vi "Get Menu Launch Info__jki_lib_application_control -- VI Tester.vi"(8 "error in (no error)":errorcluster) -> (0 "error out":errorcluster, 2 "Menu Launch info":T1)   [LabVIEW 2011]
doc: "Returns menu-launch info, including selected project items."
uses:
  Menu Launch Info - Cluster__jki_lib_application_control -- VI Tester.ctl
  Project Item Info - Cluster__jki_lib_application_control -- VI Tester.ctl
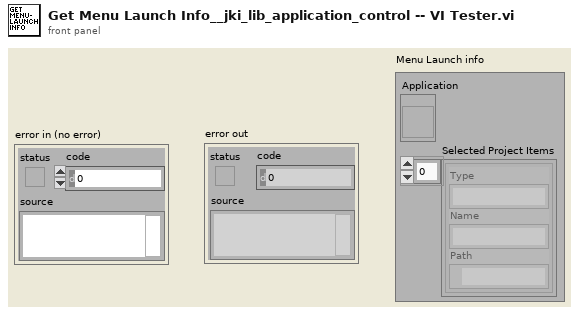
[diagram p1: front panel]
types:
  T1 = typedef "Menu Launch Info - Cluster__jki_lib_application_control -- VI Tester.ctl" = cluster{"Application":refnum<vi>, "Selected Project Items":T2[]}
  T2 = typedef "Project Item Info - Cluster__jki_lib_application_control -- VI Tester.ctl" = cluster{"Type":string, "Name":string, "Path":path}
  T3 = cluster{"App.DefaultApplication":refnum<vi>, "Selected Project Items":T2[]}
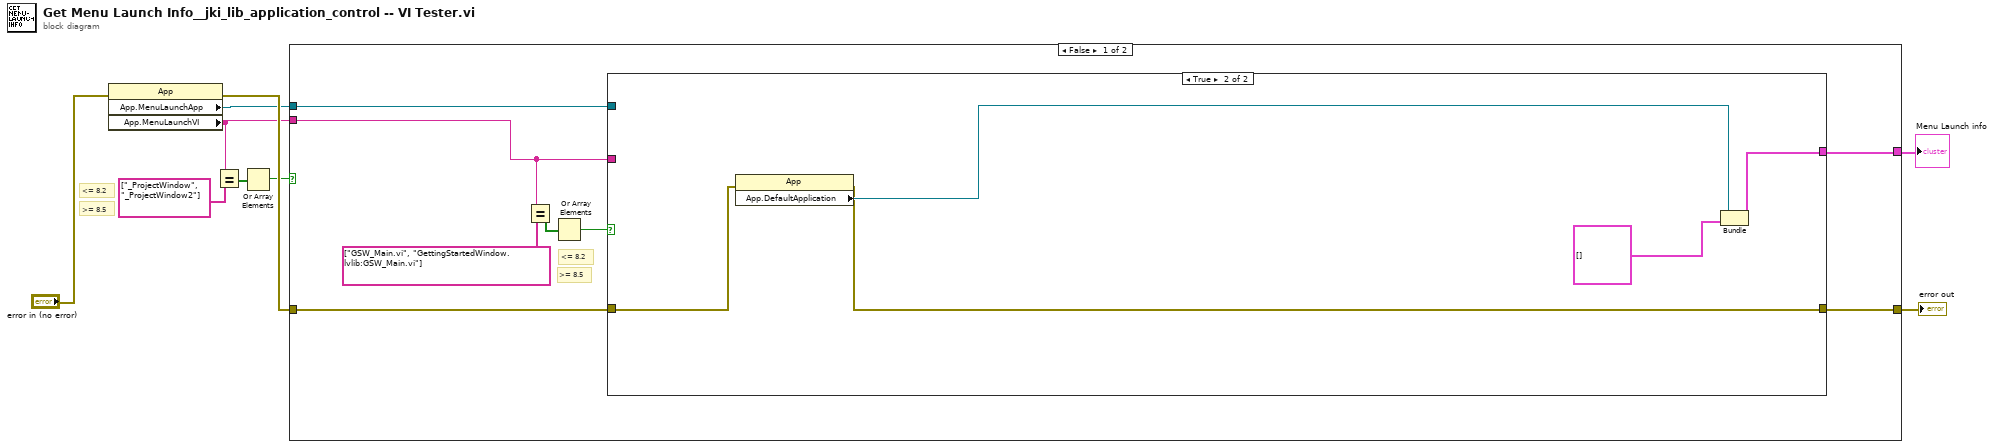
[diagram p0: block diagram]
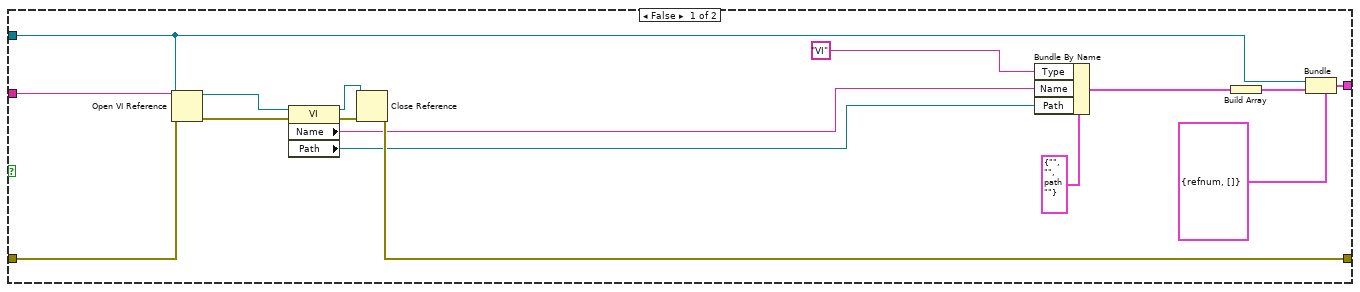
[diagram p2: hidden frame]
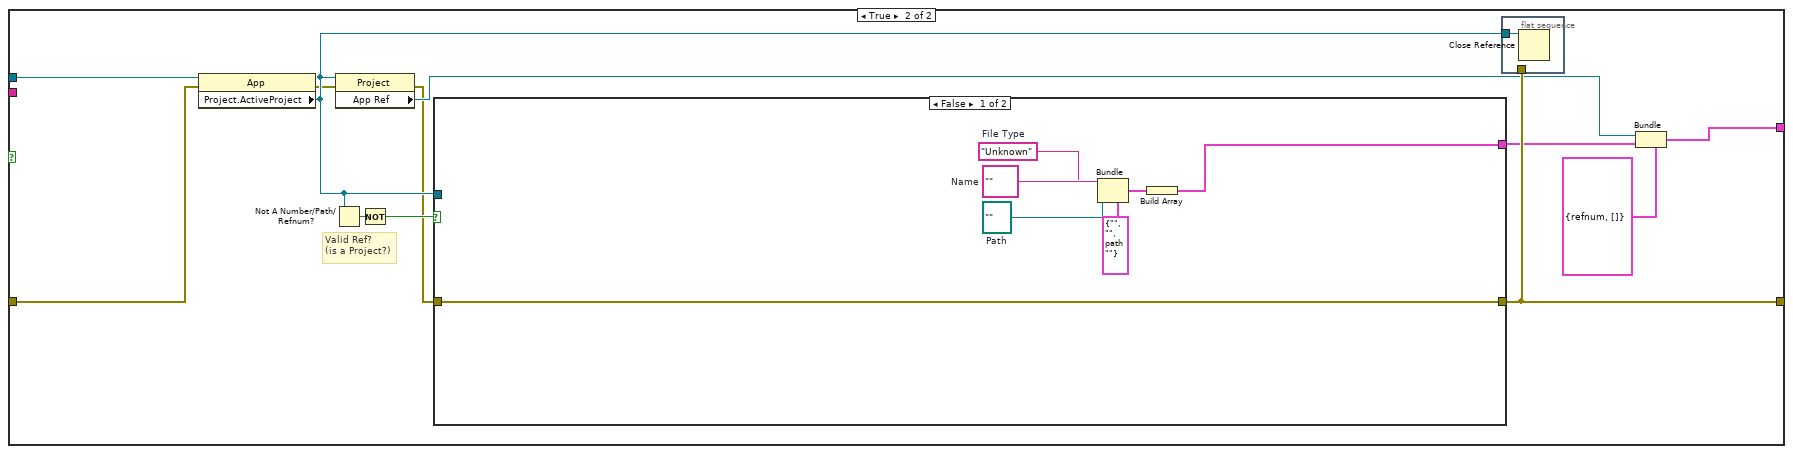
[diagram p3: hidden frame]
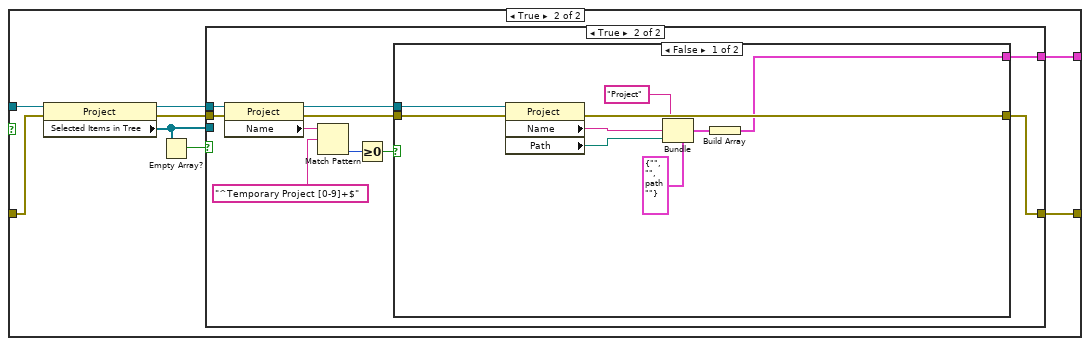
[diagram p4: hidden frame]
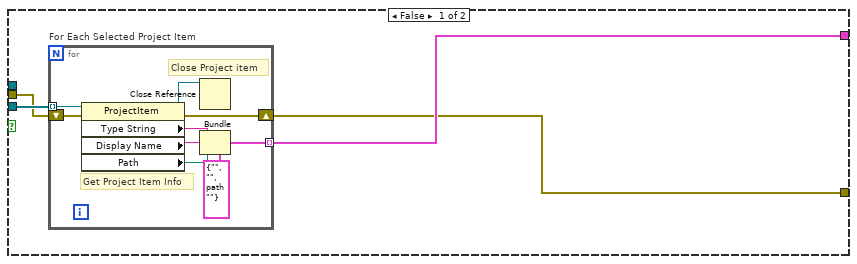
[diagram p5: hidden frame]
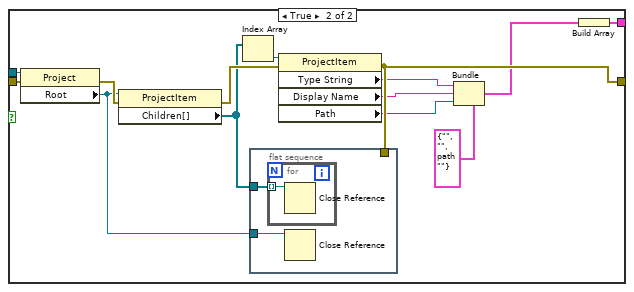
[diagram p6: hidden frame]
diagram:
  # "<= 8.2"
  # ">= 8.5"
  n1 = property class="App"(error in="error in (no error)") -> (error out=w9:errorcluster, "App.MenuLaunchApp"=w8:refnum<vi>, "App.MenuLaunchVI"=w4:string)  [unwired: 1 in, 1 out]
  n2 = Equal?(x=w4, y=string[] ["_ProjectWindow", "_ProjectWindow2"]) -> (x = y?=w2:bool[])
  n3 = Or Array Elements(Boolean array=w2) -> (logical OR=w1:bool)
  n4 = case shown="False" w1 {
    tunnel: w9 -> [w17 w50]
    tunnel: w8 -> [w15 w49]
    tunnel: [w14 w44] -> w7
    tunnel: [w16 w46] -> w6
    tunnel: w4 -> [w13 _]
    frame False {
      # "<= 8.2"
      # ">= 8.5"
      n5 = Equal?(x=w13, y=string[] ["GSW_Main.vi", "GettingStartedWindow.lvlib:GSW_Main.vi"]) -> (x = y?=w12:bool[])
      n6 = Or Array Elements(Boolean array=w12) -> (logical OR=w10:bool)
      n7 = case shown="True" w10 {
        tunnel: w17 -> [w29 w36]
        tunnel: [w28 w35] -> w16
        tunnel: w15 -> [w26 _]
        tunnel: [w25 w38] -> w14
        tunnel: w13 -> [w22 _]
        frame False {
          n8 = Open VI Reference(application reference (local)=w26, vi path=w22, error in (no error)=w29) -> (vi reference=w32:refnum<vi>, error out=w33:errorcluster)  [unwired: 3 in]
          n9 = property class="VI"(reference=w32, error in=w33) -> (reference out=w31:refnum<vi>, error out=w30:errorcluster, "Name"=w21:string, "Path"=w24:path)
          n10 = Close Reference(reference=w31, error in (no error)=w30) -> (error out=w28:errorcluster)
          n11 = Bundle By Name(cluster=T2 {"Type"="", "Name"="", "Path"=path ""} ("Project Item"), "Type"="VI" ("File Type"), "Name"=w21, "Path"=w24) -> (w23:T2)
          n12 = Build Array(w23) -> (w27:T2[])
          n13 = Bundle(cluster=T1 {"Application"=refnum, "Selected Project Items"=[]} ("Menu Launch info"), "Application"=w26, "Selected Project Items"=w27) -> (w25:T1)
        }
        frame True {
          n14 = property class="App"(error in=w36) -> (error out=w35:errorcluster, "App.DefaultApplication"=w37:refnum<vi>)  [unwired: 1 in, 1 out]
          n15 = Bundle("App.DefaultApplication"=w37, "Selected Project Items"=T2[] []) -> (w38:T3)  [unwired: 1 in]
        }
      }
    }
    frame True {
      # "Valid Ref?\n(is a Project?)"
      n16 = property class="App"(reference=w49, error in=w50) -> (error out=w41:errorcluster, "Project.ActiveProject"=w43:refnum<vi>)  [unwired: 1 out]
      n17 = Not A Number/Path/Refnum?(number/path/refnum=w43) -> (NaN/Path/Refnum?=w48:bool)
      n18 = property class="Project"(reference=w43, error in=w41) -> (error out=w40:errorcluster, "App Ref"=w42:refnum<vi>)  [unwired: 1 out]
      n19 = Not(x=w48) -> (.not. x?=w47:bool)
      n20 = case shown="False" w47 {
        tunnel: w40 -> [w58 w61]
        tunnel: w43 -> [_ w64]
        tunnel: [w58 w66] -> w46
        tunnel: [w57 w65] -> w45
        frame False {
          w56 = path ""  # Path
          w54 = ""  # Name
          w53 = "Unknown"  # File Type
          n21 = Bundle(cluster=T2 {"Type"="", "Name"="", "Path"=path ""} ("Project Item"), "Type"=w53, "Name"=w54, "Path"=w56) -> (w55:T2)
          n22 = Build Array(w55) -> (w57:T2[])
        }
        frame True {
          n23 = property class="Project"(reference=w64, error in=w61) -> (reference out=w63:refnum<vi>, error out=w62:errorcluster, "Selected Items in Tree"=w59:refnum<vi>[])
          n24 = Empty Array?(array=w59) -> (empty?=w60:bool)
          n25 = case shown="True" w60 {
            tunnel: [w67 w83] -> w66
            tunnel: [w68 w82] -> w65
            tunnel: w63 -> [_ w81]
            tunnel: w62 -> [w69 w80]
            tunnel: w59 -> [w70 _]
            frame False {
              n26 = for "For Each Selected Project Item" {
                tunnel: w70 -> [w79] mode=indexing
                tunnel: [w75] -> w68 mode=indexing
                shift-right: [w74] -> w67
                shift-left: w69 -> [w73]
                # "Close Project item"
                # "Get Project Item Info"
                n27 = property class="ProjectItem"(reference=w79, error in=w73) -> (reference out=w72:refnum<vi>, error out=w74:errorcluster, "Type String"=w78:string, "Display Name"=w77:string, "Path"=w76:path)
                n28 = Close Reference(reference=w72) -> ()  [unwired: 1 in, 1 out]
                n29 = Bundle(cluster=T2 {"Type"="", "Name"="", "Path"=path ""} ("Project Item"), "Type"=w78, "Name"=w77, "Path"=w76) -> (w75:T2)
              }
            }
            frame True {
              n30 = property class="Project"(reference=w81, error in=w80) -> (reference out=w85:refnum<vi>, error out=w84:errorcluster, "Name"=w88:string)
              n31 = Match Pattern(string=w88, regular expression="^Temporary Project [0-9]+$") -> (offset past match=w87:i32)  [unwired: 1 in, 3 out]
              n32 = Greater Or Equal To 0?(x=w87) -> (x >= 0?=w86:bool)
              n33 = case shown="False" w86 {
                tunnel: w85 -> [w98 w112]
                tunnel: w84 -> [w97 w111]
                tunnel: [w96 w107] -> w83
                tunnel: [w93 w104] -> w82
                frame False {
                  n34 = property class="Project"(reference=w98, error in=w97) -> (error out=w96:errorcluster, "Name"=w92:string, "Path"=w95:path)  [unwired: 1 out]
                  n35 = Bundle(cluster=T2 {"Type"="", "Name"="", "Path"=path ""} ("Project Item"), "Type"="Project" ("File Type"), "Name"=w92, "Path"=w95) -> (w94:T2)
                  n36 = Build Array(w94) -> (w93:T2[])
                }
                frame True {
                  n37 = property class="Project"(reference=w112, error in=w111) -> (error out=w108:errorcluster, "Root"=w105:refnum<vi>)  [unwired: 1 out]
                  n38 = property class="ProjectItem"(reference=w105, error in=w108) -> (error out=w109:errorcluster, "Children[]"=w106:refnum<vi>[])  [unwired: 1 out]
                  n39 = Index Array(array=w106) -> (element=w110:refnum<vi>)  [unwired: 1 in]
                  n40 = flat-sequence {
                    tunnel: w107 -> [_]
                    tunnel: w106 -> [w114]
                    tunnel: w105 -> [w113]
                    frame #0 {
                      n41 = for {
                        tunnel: w114 -> [w115] mode=indexing
                        n42 = Close Reference(reference=w115) -> ()  [unwired: 1 in, 1 out]
                      }
                      n43 = Close Reference(reference=w113) -> ()  [unwired: 1 in, 1 out]
                    }
                  }
                  n44 = property class="ProjectItem"(reference=w110, error in=w109) -> (error out=w107:errorcluster, "Type String"=w103:string, "Display Name"=w102:string, "Path"=w101:path)  [unwired: 1 out]
                  n45 = Bundle(cluster=T2 {"Type"="", "Name"="", "Path"=path ""} ("Project Item"), "Type"=w103, "Name"=w102, "Path"=w101) -> (w100:T2)
                  n46 = Build Array(w100) -> (w104:T2[])
                }
              }
            }
          }
        }
      }
      n47 = flat-sequence {
        tunnel: w43 -> [w51]
        tunnel: w46 -> [_]
        frame #0 {
          n48 = Close Reference(reference=w51) -> ()  [unwired: 1 in, 1 out]
        }
      }
      n49 = Bundle(cluster=T1 {"Application"=refnum, "Selected Project Items"=[]} ("Menu Launch info"), "Application"=w42, "Selected Project Items"=w45) -> (w44:T1)
    }
  }
  "error out" <- w6
  "Menu Launch info" <- w7
